vi "f9p_log_playback.vi"() -> ()   [LabVIEW 2019]
panel:
  out "2D Picture 2":picture
  out "XY 그래프":cluster{"X":dbl, "Y":dbl}[](graph)
  in  "확인 버튼":bool
  in  "path":path=path "C:/AGV/Log/07_F9P/Log_2020-07-25 home-F9P_log-4_GNGGA.txt"
  out "heading":dbl=227.42
  out "LatLong_GNRMC":cluster{dbl, dbl}={4531062.892730074, 6178443.004085811} {"?" format="%.11f"; "?" format="%.11f"}
  out "str_GNRMC":string="065308.00,A,3723.59854,N,12656.92439,E,0.023,,250720,,,A,V*1C"
  out "str-arr_GNRMC":string[](array[string])=["065308.00", "A", "3723.59854", "N", "12656.92439", "E", "0.023", "", "250720", "", "", "A", "V*1C"]
  out "GNRMC_val":bool
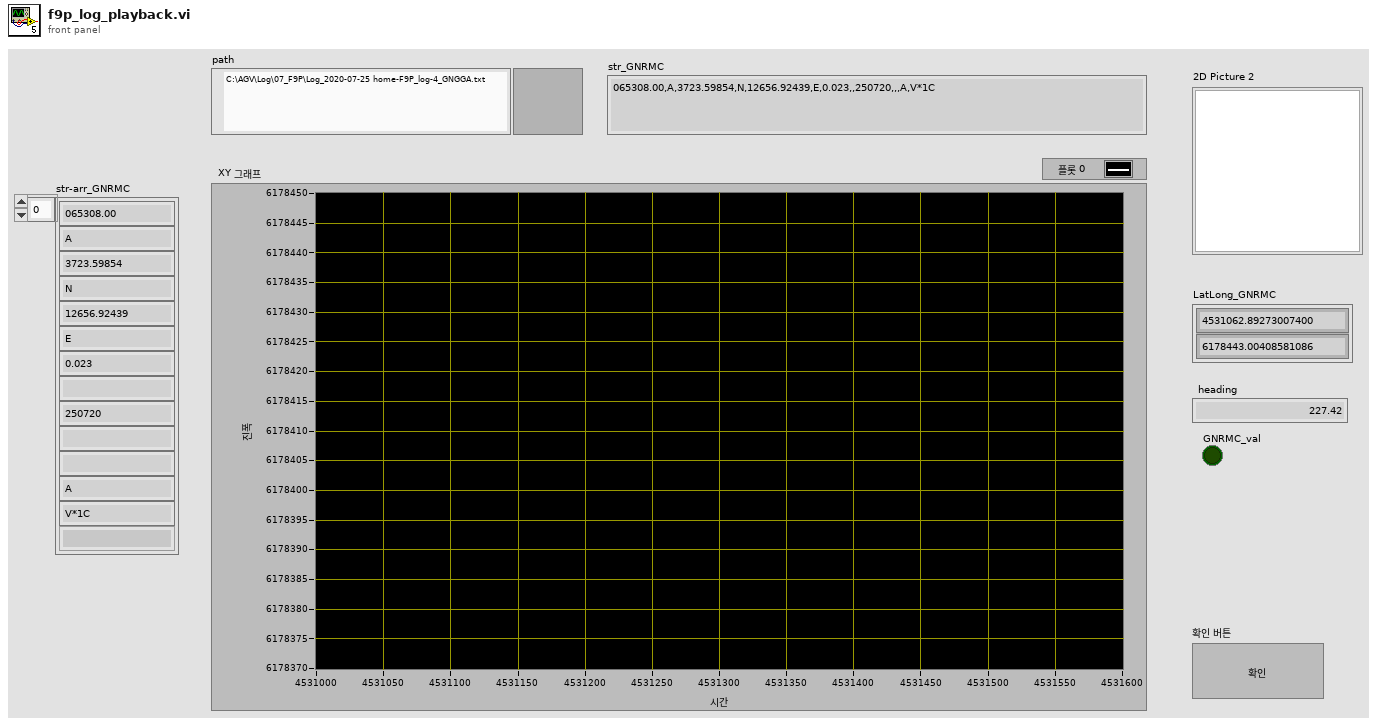
[diagram p1: front panel]
types:
  T1 = enum16{"open", "replace", "create", "open or create", "replace or create", "replace or create with confirmation"}
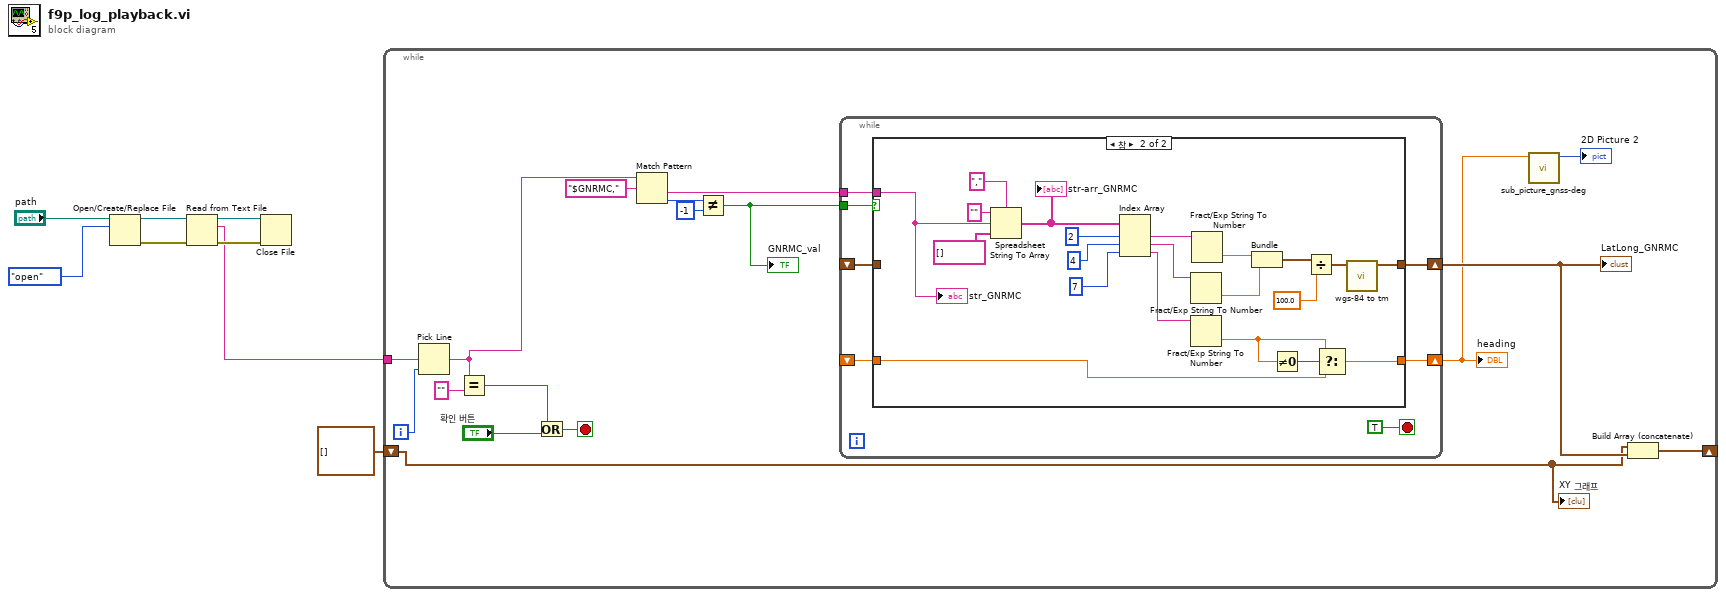
[diagram p0: block diagram]
diagram:
  n1 = Open/Create/Replace File(file path (use dialog)="path", operation (0:open)=T1."open" ("동작(0:open)")) -> (refnum out=w8:refnum<file>, error out=w5:errorcluster)  [unwired: 4 in, 1 out]
  n2 = Read from Text File(file (use dialog)=w8, error in=w5) -> (refnum out=w7:refnum<file>, text=w2:string, error out=w6:errorcluster)  [unwired: 2 in, 1 out]
  n3 = Close File(refnum=w7, error in=w6) -> ()  [unwired: 2 out]
  n4 = while {
    tunnel: w2 -> [w25]
    shift-right: [w14] -> _
    shift-left: cluster{"Y(E)":dbl, "X(N)":dbl}[] [] -> [w12]
    i -> [w24]
    stop <- w20 stop-if-true
    n5 = Pick Line(multi-line string=w25, line index=w24) -> (output string=w11:string)  [unwired: 1 in]
    n6 = Equal?(x=w11, y="") -> (x = y?=w21:bool)
    n7 = Or(x=w21, y="확인 버튼") -> (x .or. y?=w20:bool)
    n8 = Match Pattern(string=w11, regular expression="$GNRMC," ("정규식")) -> (after substring=w17:string, offset past match=w19:i32)  [unwired: 1 in, 2 out]
    n9 = Not Equal?(x=w19, y=-1) -> (x != y?=w18:bool)
    "GNRMC_val" <- w18
    n10 = while {
      tunnel: w18 -> [w32]
      tunnel: w17 -> [w31]
      shift-right: [w29] -> w13
      shift-left: _ -> [w28]
      shift-right: [w27] -> w9
      shift-left: _ -> [w26]
      stop <- TRUE stop-if-true
      n11 = case shown="참" w32 {
        tunnel: w31 -> [_ w43]
        tunnel: [w34 w39] -> w29
        tunnel: w28 -> [w34 _]
        tunnel: [w33 w35] -> w27
        tunnel: w26 -> [w33 w36]
        frame False {
        }
        frame True {
          n12 = Spreadsheet String To Array(delimiter (Tab)="," ("구분 문자 (탭)"), format string="" ("포맷 문자열"), spreadsheet string=w43, array type (2D Dbl)=string[] []) -> (array=w47:string[])
          "str-arr_GNRMC" <- w47
          n13 = Index Array(array=w47, index #1=2 ("인덱스"), index #2=4 ("인덱스"), index #3=7 ("인덱스")) -> (element #1=w50:string, element #2=w51:string, element #3=w41:string)
          n14 = Fract/Exp String To Number(string=w51) -> (number=w53:dbl)  [unwired: 3 in, 1 out]
          n15 = Fract/Exp String To Number(string=w41) -> (number=w37:dbl)  [unwired: 3 in, 1 out]
          n16 = Fract/Exp String To Number(string=w50) -> (number=w52:dbl)  [unwired: 3 in, 1 out]
          n17 = Bundle(w52, w53) -> (w55:cluster{dbl, dbl})  [unwired: 1 in]
          n18 = Not Equal To 0?(x=w37) -> (x != 0?=w38:bool)
          n19 = Divide(x=w55, y=100.0) -> (x/y=w40:cluster{dbl, dbl})
          n20 = Select(t=w37, s=w38, f=w36) -> (s? t:f=w35:dbl)
          n21 = call "wgs-84 to tm.vi"("in_lon-lat"=w40) -> ("TM"=w39:cluster{"Y(E)":dbl, "X(N)":dbl})  [unwired: 10 in]
          "str_GNRMC" <- w43
        }
      }
    }
    "LatLong_GNRMC" <- w13
    "heading" <- w9
    n22 = call "sub_picture_gnss-deg.vi"("deg_gps"=w9) -> ("new picture"=→"2D Picture 2":picture)  [unwired: 10 in]
    n23 = Build Array (concatenate)(w12, w13) -> (w14:cluster{"Y(E)":dbl, "X(N)":dbl}[])
    "XY 그래프" <- w12
  }
